vi "בדיקת מתח שחרור של סליל פיקוד ללא עומס 5.vi"(7 "userResult":bool=TRUE, 8 "error":errorcluster, 10 "lines":tag="PXI1Slot8/port0/line1", 11 "Path for Log":path) -> (0 "error out":errorcluster, 1 "מצב ממסר פתוח/סגור":bool, 2 "מתח פתיחת הממסר":dbl format="%.4f", 3 "מתח מוצא מהספק":dbl format="%.4f")   [LabVIEW 2014]
uses:
  <vilib>/DAQmx/create/channels.llb/DAQmx Create Channel (DO-Digital Output).vi
  <vilib>/DAQmx/write.llb/DAQmx Write (Digital Bool 1Line 1Point).vi
panel:
  out "progress":dbl(slide) scale=0.0..11.0
  out "error IO DMM":errorcluster
  in  "Stop Button":bool
  # "Right-Click to\nexplain error"
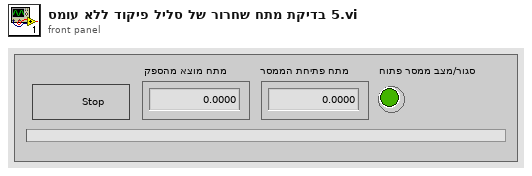
[diagram p1: front panel]
types:
  T1 = enum32{"Invalid", "Standard", "Closed", "Hidden", "Minimized", "Maximized"}
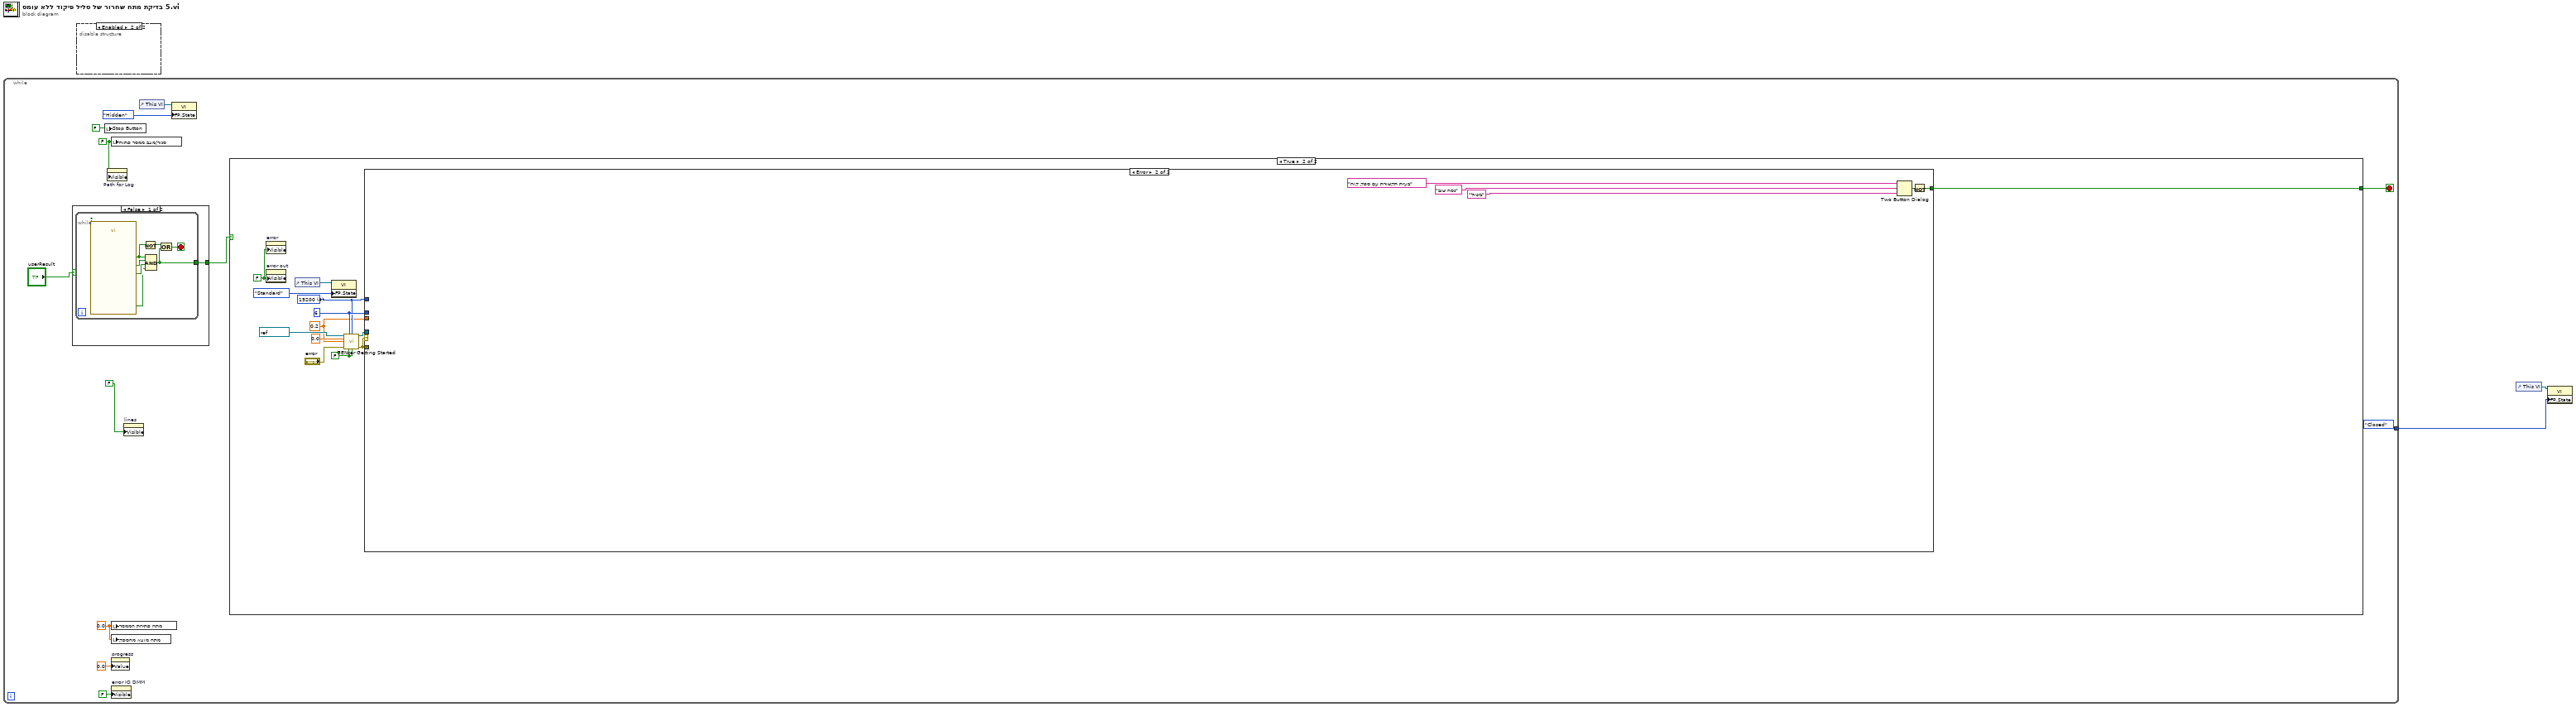
[diagram p0: block diagram]
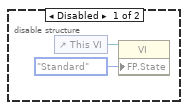
[diagram p2: hidden frame]
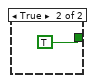
[diagram p3: hidden frame]
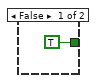
[diagram p4: hidden frame]
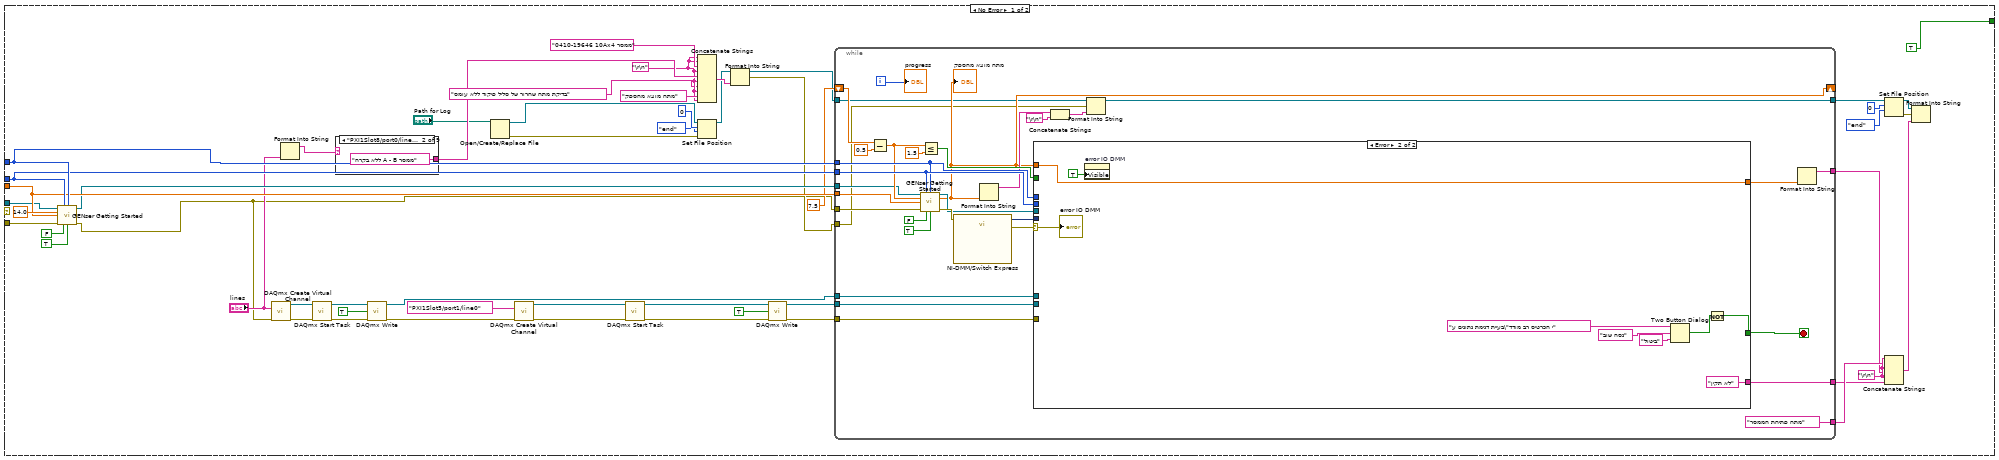
[diagram p5: hidden frame]
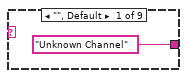
[diagram p6: hidden frame]
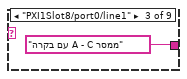
[diagram p7: hidden frame]
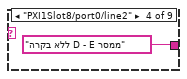
[diagram p8: hidden frame]
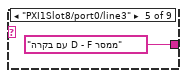
[diagram p9: hidden frame]
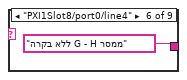
[diagram p10: hidden frame]
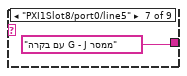
[diagram p11: hidden frame]
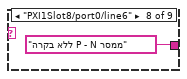
[diagram p12: hidden frame]
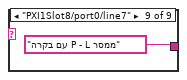
[diagram p13: hidden frame]
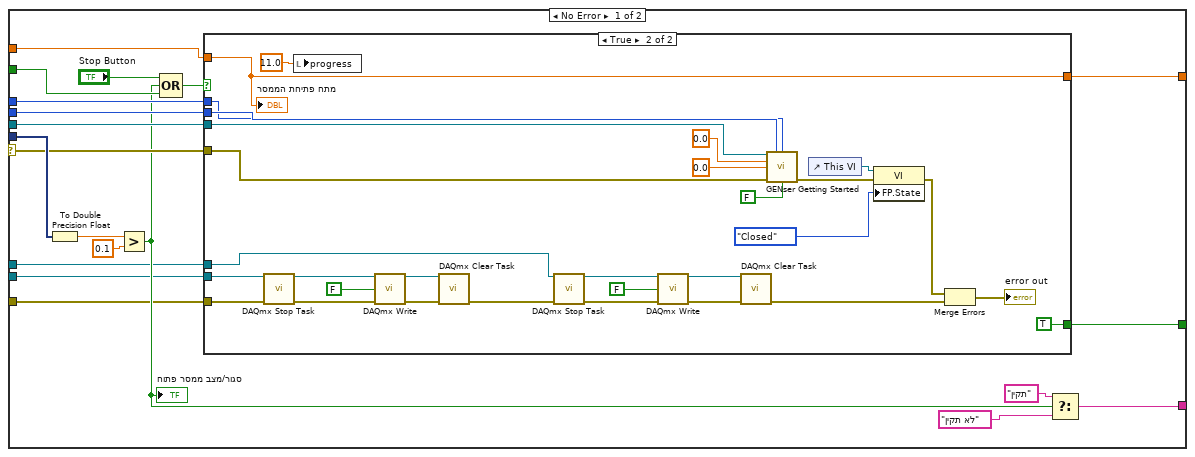
[diagram p14: hidden frame]
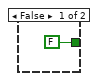
[diagram p15: hidden frame]
diagram:
  n1 = while {
    tunnel: [T1."Closed" ("Front Panel Window:State")] -> w1
    stop <- w5 stop-if-true
    w8 = FALSE ("מגע סגור")
    w11 = 0.0 ("signals out")
    n2 = case shown="False" "userResult" {
      tunnel: [w15 TRUE] -> w7
      frame False {
        n3 = while {
          tunnel: [w16] -> w15
          stop <- w19 stop-if-true
          n4 = call "?"() -> ("הדקי הרב מודד"=w20:bool, "M מגע שלילי"=w21:bool, "K מגע חיובי"=w22:bool, "OK"=w17:bool)  [unwired: 15 in, 1 out]
          n5 = Not(x=w17) -> (.not. x?=w18:bool)
          n6 = Compound Arithmetic op=AND(w17, w22, w21, w20) -> (w16:bool)
          n7 = Or(x=w18, y=w16) -> (x .or. y?=w19:bool)
        }
      }
      frame True {
      }
    }
    n8 = local write "Stop Button"(FALSE ("Reset (T)")) -> ()
    n9 = property on="Path for Log" class="Path"("Visible"=w8) -> ()  [unwired: 2 in, 2 out]
    n10 = local write "מצב ממסר פתוח/סגור"(w8) -> ()
    n11 = local write "מתח פתיחת הממסר"(w11) -> ()
    n12 = local write "מתח מוצא מהספק"(w11) -> ()
    n13 = property on="progress" class="Slide (strict)"("Value"=0.0 ("progress")) -> ()  [unwired: 2 in, 2 out]
    n14 = property on="error IO DMM" class="Clust (strict)"("Visible"=FALSE) -> ()  [unwired: 2 in, 2 out]
    n15 = property on="lines" class="DAQmxName"("Visible"=FALSE) -> ()  [unwired: 2 in, 2 out]
    n16 = control-ref of="This VI"() -> (w10:refnum<vi>)
    n17 = property class="VI"(reference=w10, "FP.State"=T1."Hidden" ("Front Panel Window:State")) -> ()  [unwired: 1 in, 2 out]
    n18 = case shown="True" w7 {
      tunnel: [TRUE ("T button?") w29] -> w5
      frame False {
      }
      frame True {
        w27 = FALSE ("Visible")
        w28 = FALSE ("Output On (T)")
        w33 = u16 4 items=["1200", "2400", "4800", "9600", "19200"] ("BAUD")
        w34 = i16 6 ("GEN Addr")
        w30 = 0.2 ("Current Limit")
        n19 = property on="error" class="Clust (strict)"("Visible"=w27) -> ()  [unwired: 2 in, 2 out]
        n20 = property on="error out" class="Clust (strict)"("Visible"=w27) -> ()  [unwired: 2 in, 2 out]
        n21 = control-ref of="This VI"() -> (w25:refnum<vi>)
        n22 = property class="VI"(reference=w25, "FP.State"=T1."Standard" ("Front Panel Window:State")) -> ()  [unwired: 1 in, 2 out]
        n23 = call "GENser Getting Started.vi"("VISA"=refnum<visa-resource-name> "COM6", "GEN Addr"=w34, "BAUD"=w33, "Voltage Limit"=0.0, "Current Limit"=w30, "error"="error", "Reset (T)"=w28, "Output On (T)"=w28) -> ("VISA out"=w35:refnum<visa-resource-name>, "error out"=w36:errorcluster)  [unwired: 4 in, 2 out]
        n24 = case shown="Error" w36 {
          tunnel: w36 -> [w87 _]
          tunnel: w35 -> [w83 _]
          tunnel: w34 -> [w85 _]
          tunnel: w33 -> [w86 _]
          tunnel: w30 -> [w84 _]
          tunnel: [TRUE w192] -> w29
          frame No Error {
            w44 = "\r\n"
            w79 = "\r\n"
            n25 = call "GENser Getting Started.vi"("VISA"=w83, "GEN Addr"=w85, "BAUD"=w86, "Voltage Limit"=14.0, "Current Limit"=w84, "error"=w87, "Reset (T)"=FALSE, "Output On (T)"=TRUE) -> ("VISA out"=w82:refnum<visa-resource-name>, "error out"=w38:errorcluster)  [unwired: 4 in, 2 out]
            n26 = call-poly <vilib>:"DAQmx Create Virtual Channel.vi"("lines"="lines", "error in"=w38) -> ("task out"=w61:refnum<k21>, "error out"=w60:errorcluster)  [unwired: 12 in]
            n27 = Format Into String("lines") -> (resulting string=w47:string)  [unwired: 3 in, 1 out]
            n28 = call <vilib>:"DAQmx Start Task.vi"("task/channels in"=w61, "error in"=w60) -> ("task out"=w58:refnum<k21>, "error out"=w59:errorcluster)  [unwired: 12 in]
            n29 = case shown="\"PXI1Slot8/port0/line0\"" w47 {
              tunnel: ["Unknown Channel" "ללא בקרה A - B ממסר" "עם בקרה A - C ממסר" "ללא בקרה D - E ממסר" "עם בקרה D - F ממסר" "ללא בקרה G - H ממסר" "עם בקרה G - J ממסר" "ללא בקרה P - N ממסר" "עם בקרה P - L ממסר"] -> w46
              frame "", Default {
              }
              frame "PXI1Slot8/port0/line0" {
              }
              frame "PXI1Slot8/port0/line1" {
              }
              frame "PXI1Slot8/port0/line2" {
              }
              frame "PXI1Slot8/port0/line3" {
              }
              frame "PXI1Slot8/port0/line4" {
              }
              frame "PXI1Slot8/port0/line5" {
              }
              frame "PXI1Slot8/port0/line6" {
              }
              frame "PXI1Slot8/port0/line7" {
              }
            }
            n30 = call-poly <vilib>:"DAQmx Write.vi"("task/channels in"=w58, "data"=TRUE, "error in"=w59) -> ("task out"=w55:refnum<k21>, "error out"=w56:errorcluster)  [unwired: 10 in, 1 out]
            n31 = Open/Create/Replace File(file path (use dialog)="Path for Log") -> (refnum out=w52:refnum<file>, error out=w51:errorcluster)  [unwired: 5 in, 1 out]
            n32 = call-poly <vilib>:"DAQmx Create Virtual Channel.vi"("lines"=tag "PXI1Slot5/port1/line0", "error in"=w56) -> ("task out"=w68:refnum<k21>, "error out"=w69:errorcluster)  [unwired: 12 in]
            n33 = call <vilib>:"DAQmx Start Task.vi"("task/channels in"=w68, "error in"=w69) -> ("task out"=w66:refnum<k21>, "error out"=w65:errorcluster)  [unwired: 12 in]
            n34 = Concatenate Strings(w44, w44, "0410-19646 10Ax4 ממסר", w44, w46, w44, "בדיקת מתח שחרור של סליל פיקוד ללא עומס", w44, "מתח מוצא מהספק", w44) -> (w50:string)
            n35 = Set File Position(offset (in bytes) (0)=i64 0, refnum=w52, from (0:start)=enum16{"start", "end", "current"}."end", error in=w51) -> (refnum out=w48:refnum<file>)  [unwired: 1 out]
            n36 = Format Into String(initial string=w48, w50) -> (resulting string=w39:refnum<file>, error out=w40:errorcluster)  [unwired: 2 in]
            n37 = call-poly <vilib>:"DAQmx Write.vi"("task/channels in"=w66, "data"=TRUE, "error in"=w65) -> ("task out"=w63:refnum<k21>, "error out"=w62:errorcluster)  [unwired: 10 in, 1 out]
            n38 = while {
              tunnel: w38 -> [w131]
              tunnel: w85 -> [w124]
              tunnel: w86 -> [w123]
              tunnel: w84 -> [w129]
              shift-right: [w106] -> _
              shift-left: 7.5 ("y") -> [w127]
              tunnel: w82 -> [w116]
              tunnel: [w111] -> w74
              tunnel: ["מתח פתיחת הממסר"] -> w73
              tunnel: [w109] -> w72
              tunnel: [w108] -> w71
              tunnel: w39 -> [w105]
              tunnel: w40 -> [w101]
              tunnel: w63 -> [w104]
              tunnel: w62 -> [w103]
              tunnel: w55 -> [w102]
              i -> [w117]
              stop <- w100 stop-if-true
              n39 = Subtract(x=w127, y=0.5) -> (x-y=w120:dbl)
              n40 = call "GENser Getting Started.vi"("VISA"=w116, "GEN Addr"=w124, "BAUD"=w123, "Voltage Limit"=w120, "Current Limit"=w129, "error"=w131, "Reset (T)"=FALSE, "Output On (T)"=TRUE) -> ("VISA out"=w122:refnum<visa-resource-name>, "Output Voltage"=w106:dbl, "error out"=w126:errorcluster)  [unwired: 4 in, 1 out]
              "מתח מוצא מהספק" <- w106
              n41 = Less Or Equal?(x=w120, y=1.5) -> (x <= y?=w119:bool)
              n42 = call "NI-DMM/Switch Express"("error in"=w126) -> ("signals out"=w125:dynamicdata, "error out"=w118:errorcluster)  [unwired: 16 in, 1 out]
              n43 = Format Into String(w106) -> (resulting string=w113:string)  [unwired: 3 in, 1 out]
              n44 = case shown="Error" w118 {
                selector: w118 -> [w142 w191]
                tunnel: w125 -> [w151 _]
                tunnel: [w148 w183] -> w100
                tunnel: w124 -> [w147 _]
                tunnel: w123 -> [w146 _]
                tunnel: w122 -> [w145 _]
                tunnel: w119 -> [w144 _]
                tunnel: w106 -> [w143 w186]
                tunnel: [w136 w186] -> w112
                tunnel: [w135 "לא תקין"] -> w108
                tunnel: w104 -> [w134 _]
                tunnel: w103 -> [w133 _]
                tunnel: w102 -> [w132 _]
                frame No Error {
                  n45 = To Double Precision Float(number=w151) -> (double precision float=w141:dbl)
                  n46 = Greater?(x=w141, y=0.1) -> (0:w137:bool)
                  "מצב ממסר פתוח/סגור" <- w137
                  n47 = Compound Arithmetic op=OR("Stop Button", w137, w144) -> (w150:bool)
                  n48 = case shown="True" w150 {
                    tunnel: [FALSE TRUE] -> w148
                    tunnel: w147 -> [_ w181]
                    tunnel: w146 -> [_ w180]
                    tunnel: w145 -> [_ w179]
                    tunnel: w142 -> [_ w176]
                    tunnel: w143 -> [_ w170]
                    tunnel: [_ w170] -> w136
                    tunnel: w134 -> [_ w164]
                    tunnel: w133 -> [_ w163]
                    tunnel: w132 -> [_ w154]
                    frame False {
                    }
                    frame True {
                      n49 = call <vilib>:"DAQmx Stop Task.vi"("task/channels in"=w164, "error in"=w163) -> ("task out"=w169:refnum<k21>, "error out"=w168:errorcluster)  [unwired: 12 in]
                      n50 = local write "progress"(11.0 ("progress")) -> ()
                      n51 = call-poly <vilib>:"DAQmx Write.vi"("task/channels in"=w169, "data"=FALSE, "error in"=w168) -> ("task out"=w167:refnum<k21>, "error out"=w166:errorcluster)  [unwired: 10 in, 1 out]
                      n52 = call <vilib>:"DAQmx Clear Task.vi"("task in"=w167, "error in"=w166) -> ("error out"=w155:errorcluster)  [unwired: 13 in]
                      n53 = call <vilib>:"DAQmx Stop Task.vi"("task/channels in"=w154, "error in"=w155) -> ("task out"=w156:refnum<k21>, "error out"=w158:errorcluster)  [unwired: 12 in]
                      n54 = call-poly <vilib>:"DAQmx Write.vi"("task/channels in"=w156, "data"=FALSE, "error in"=w158) -> ("task out"=w159:refnum<k21>, "error out"=w160:errorcluster)  [unwired: 10 in, 1 out]
                      n55 = call <vilib>:"DAQmx Clear Task.vi"("task in"=w159, "error in"=w160) -> ("error out"=w153:errorcluster)  [unwired: 13 in]
                      n56 = call "GENser Getting Started.vi"("VISA"=w179, "GEN Addr"=w181, "BAUD"=w180, "Voltage Limit"=0.0, "Current Limit"=0.0, "error"=w176, "Output On (T)"=FALSE) -> ("error out"=w171:errorcluster)  [unwired: 5 in, 3 out]
                      n57 = control-ref of="This VI"() -> (w172:refnum<vi>)
                      n58 = property class="VI"(reference=w172, error in=w171, "FP.State"=T1."Closed" ("Front Panel Window:State")) -> (error out=w162:errorcluster)  [unwired: 1 out]
                      n59 = Merge Errors(w162, w153) -> (→"error out":errorcluster)
                      "מתח פתיחת הממסר" <- w170
                    }
                  }
                  n60 = Select(t="תקין", s=w137, f="לא תקין") -> (s? t:f=w135:string)
                }
                frame Error {
                  n61 = property on="error IO DMM" class="Clust (strict)"("Visible"=TRUE) -> ()  [unwired: 2 in, 2 out]
                  n62 = Two Button Dialog(message="בעיית דגימת נתונים ע\"י הכרטיס רב מודד", 1:"ביטול" ("F button name (\"Cancel\")"), 2:"נסה שוב" ("T button name (\"OK\")")) -> (T button?=w184:bool)
                  n63 = Not(x=w184) -> (.not. x?=w183:bool)
                  "error IO DMM" <- w191
                }
              }
              n64 = Concatenate Strings(w113, "\r\n") -> (w107:string)
              n65 = Format Into String(initial string=w105, error in=w101, w107) -> (resulting string=w111:refnum<file>)  [unwired: 1 in, 1 out]
              n66 = Format Into String(w112) -> (resulting string=w109:string)  [unwired: 3 in, 1 out]
              "progress" <- w117
            }
            n67 = Set File Position(offset (in bytes) (0)=i64 0, refnum=w74, from (0:start)=enum16{"start", "end", "current"}."end") -> (refnum out=w76:refnum<file>, error out=w75:errorcluster)  [unwired: 1 in]
            n68 = Concatenate Strings(w79, w73, w79, w72, w79, w71) -> (w70:string)
            n69 = Format Into String(initial string=w76, error in=w75, w70) -> ()  [unwired: 1 in, 2 out]
          }
          frame Error {
            n70 = Two Button Dialog(message="בעיית תקשורת עם ספק קוח", 1:"ביטול" ("F button name (\"Cancel\")"), 2:"נסה שוב" ("T button name (\"OK\")")) -> (T button?=w193:bool)
            n71 = Not(x=w193) -> (.not. x?=w192:bool)
          }
        }
      }
    }
  }
  n72 = disable-structure shown="Enabled" {
    frame Disabled {
      n73 = control-ref of="This VI"() -> (w197:refnum<vi>)
      n74 = property class="VI"(reference=w197, "FP.State"=T1."Standard" ("Front Panel Window:State")) -> ()  [unwired: 1 in, 2 out]
    }
    frame Enabled {
    }
  }
  n75 = control-ref of="This VI"() -> (w2:refnum<vi>)
  n76 = property class="VI"(reference=w2, "FP.State"=w1) -> ()  [unwired: 1 in, 2 out]
